vi "ILABs_RemotePanelHandler.vi"(2 "error In":errorcluster, 3 "appReference":refnum<vi>, 4 "data":string, 5 "action":string) -> (0 "errorOut":string, 1 "response":string)   [LabVIEW 2009]
panel:
  in  "Case Constant\n(See Context Help)":bool=TRUE
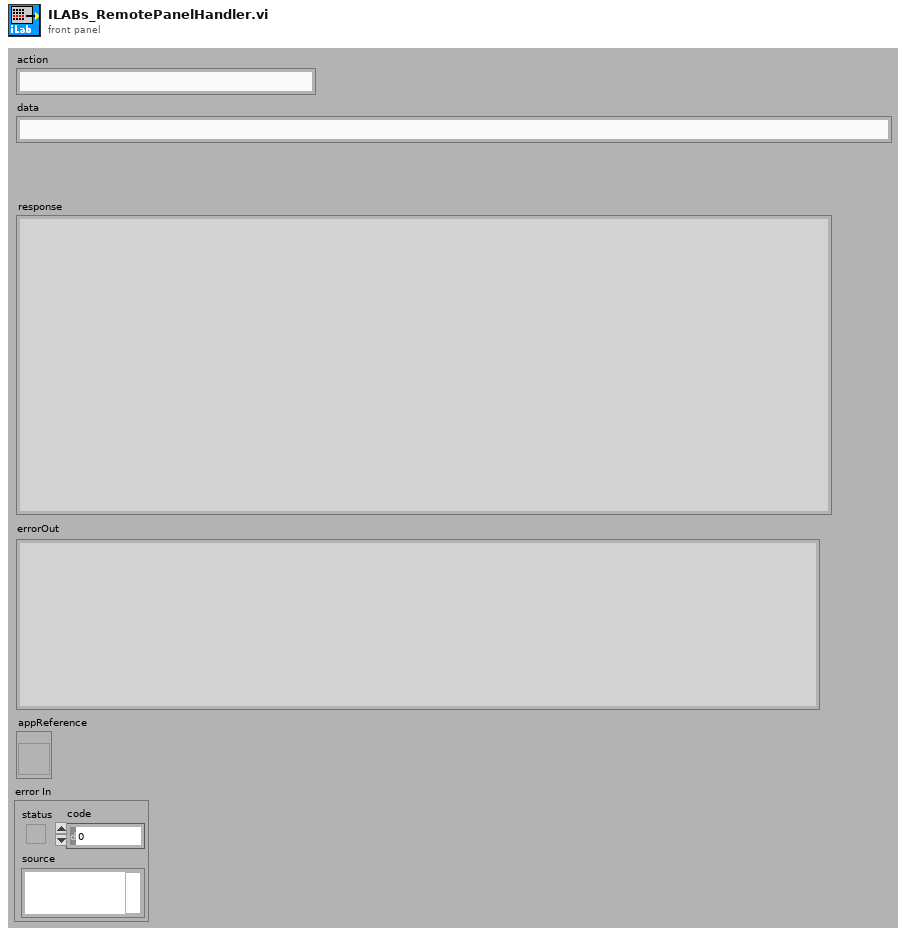
[diagram p1: front panel]
types:
  T1 = enum32{"Bad", "Idle", "Run top level", "Running"}
  T2 = typedef "LVRemotePanelConnectionsTypeDef.ctl" = cluster{"VI Name":string, "Remote":string, "UserName":string, "Port":i32, "Status":enum32{"Viewing", "Waiting For Control", "Controlling"}, "Create Time":timestamp, "Status Time":timestamp, "Control End Time":timestamp}[]
  T3 = cluster{"VI Name":string, "Remote":string, "UserName":string, "Port":i32, "Status":enum32{"Viewing", "Waiting For Control", "Controlling"}, "Create Time":timestamp, "Status Time":timestamp, "Control End Time":timestamp}
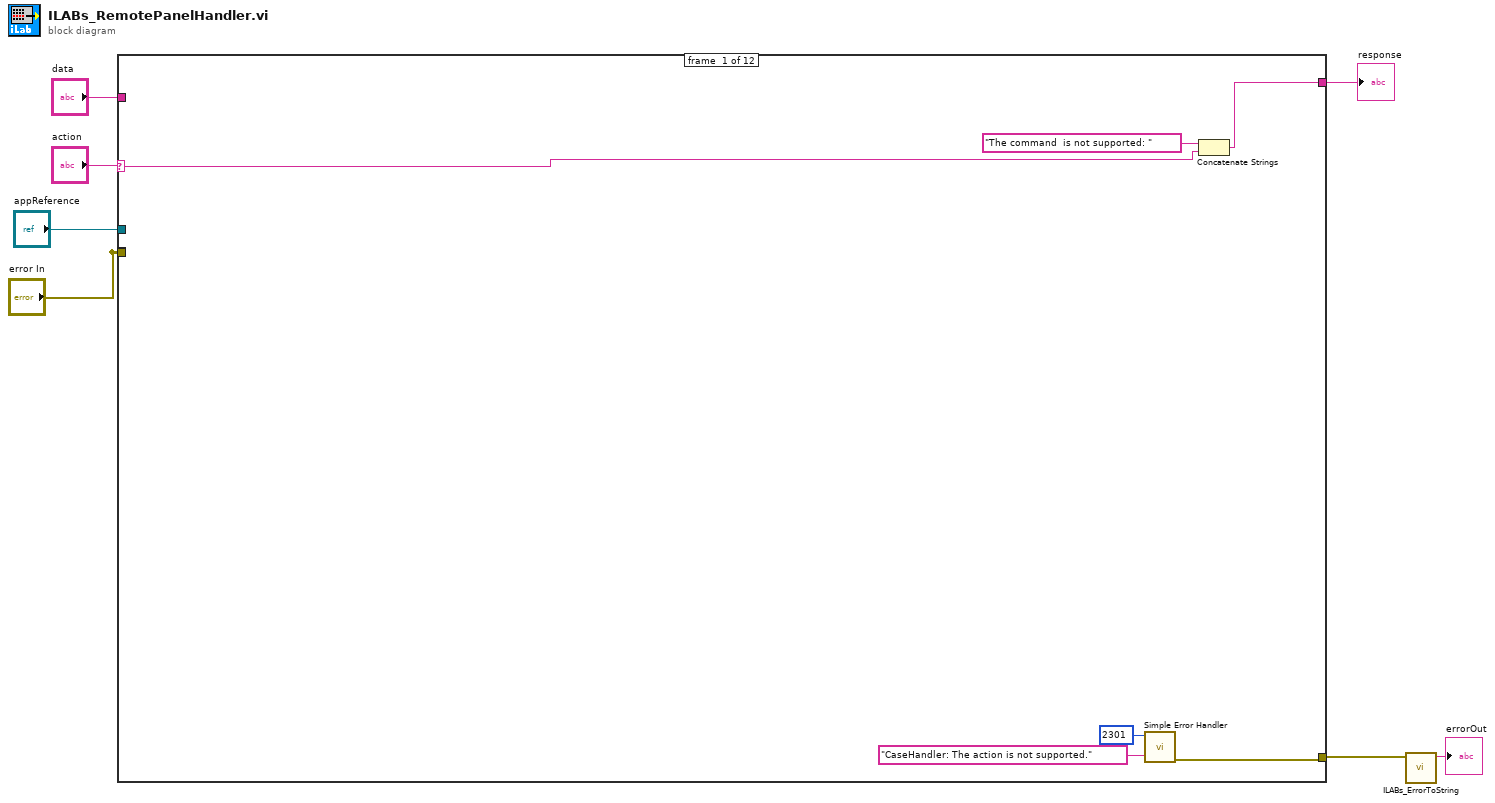
[diagram p0: block diagram]
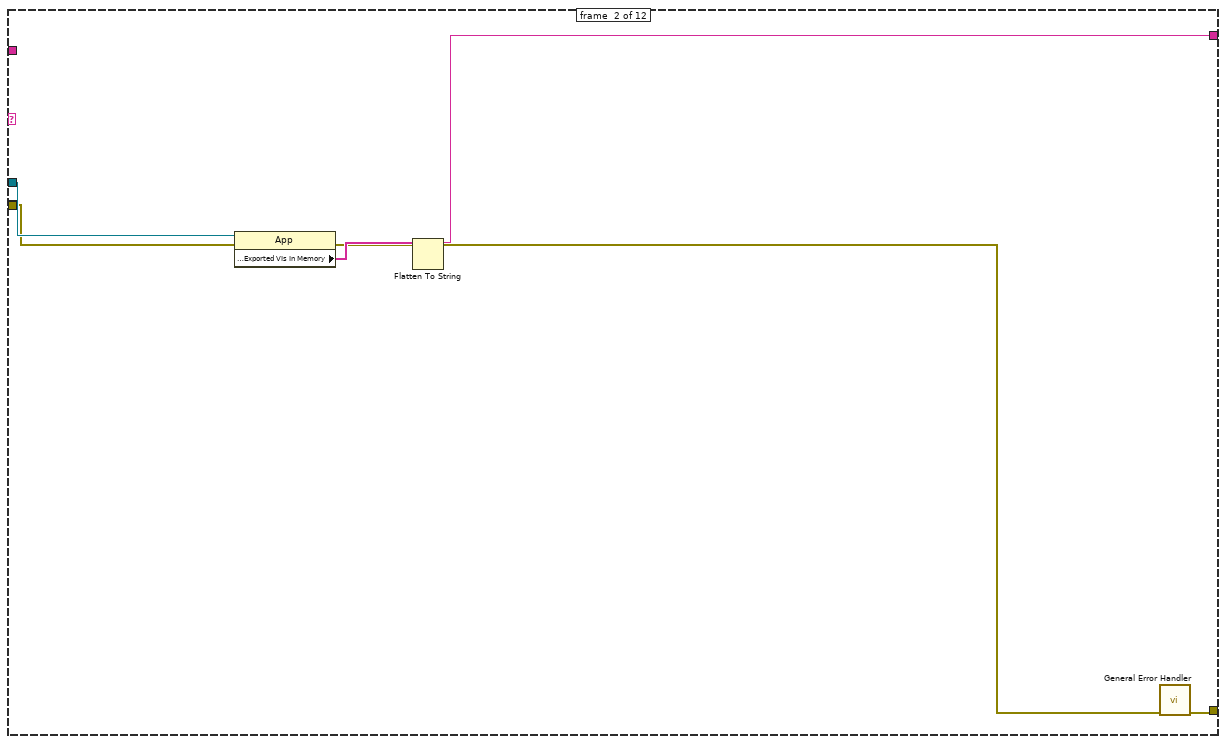
[diagram p2: hidden frame]
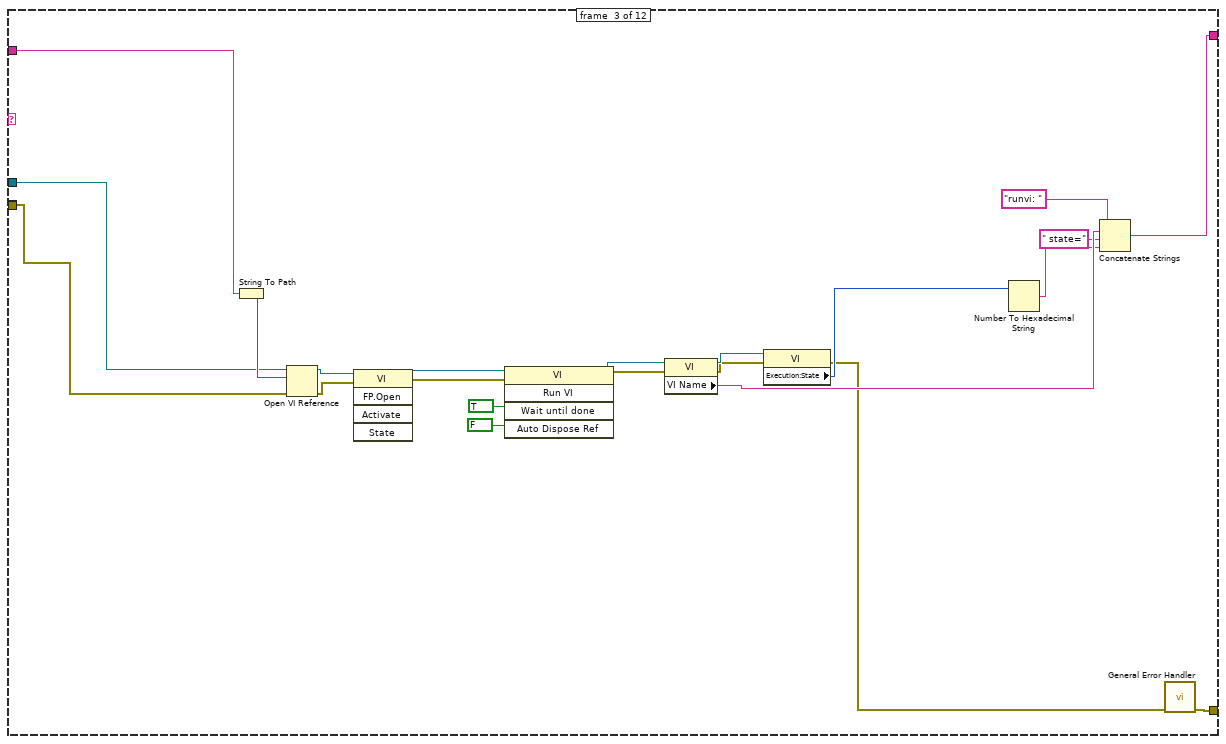
[diagram p3: hidden frame]
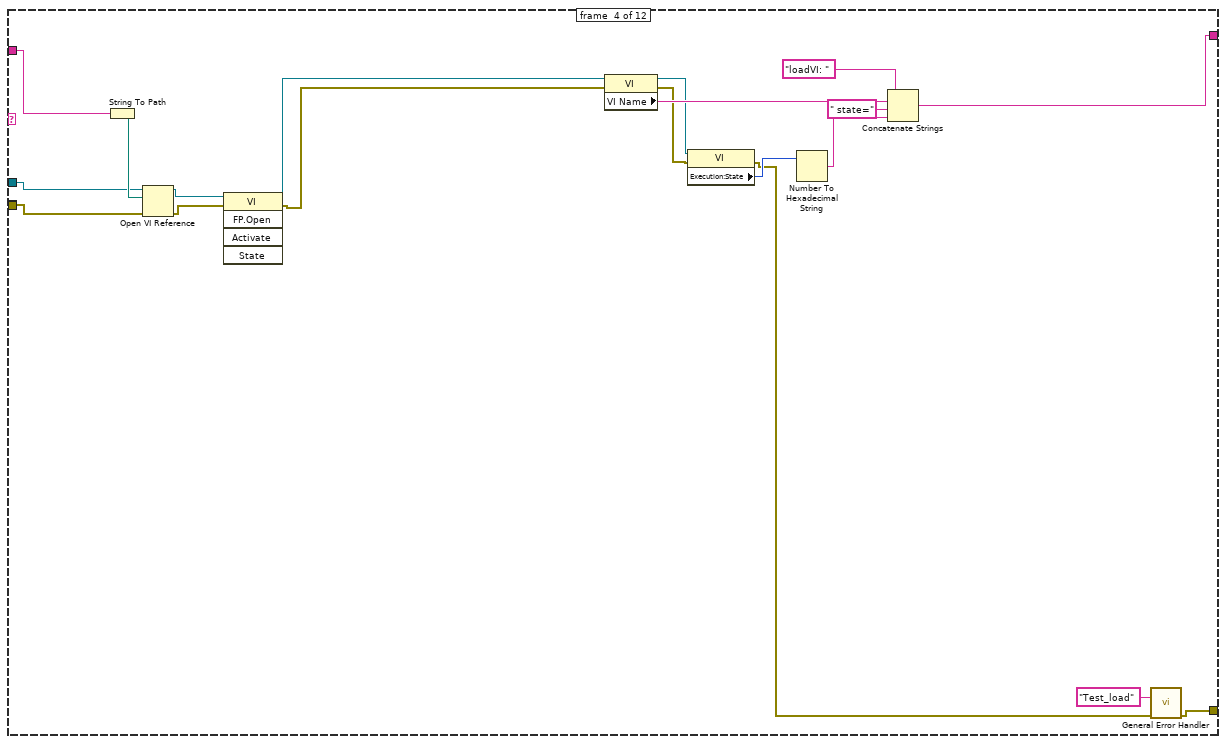
[diagram p4: hidden frame]
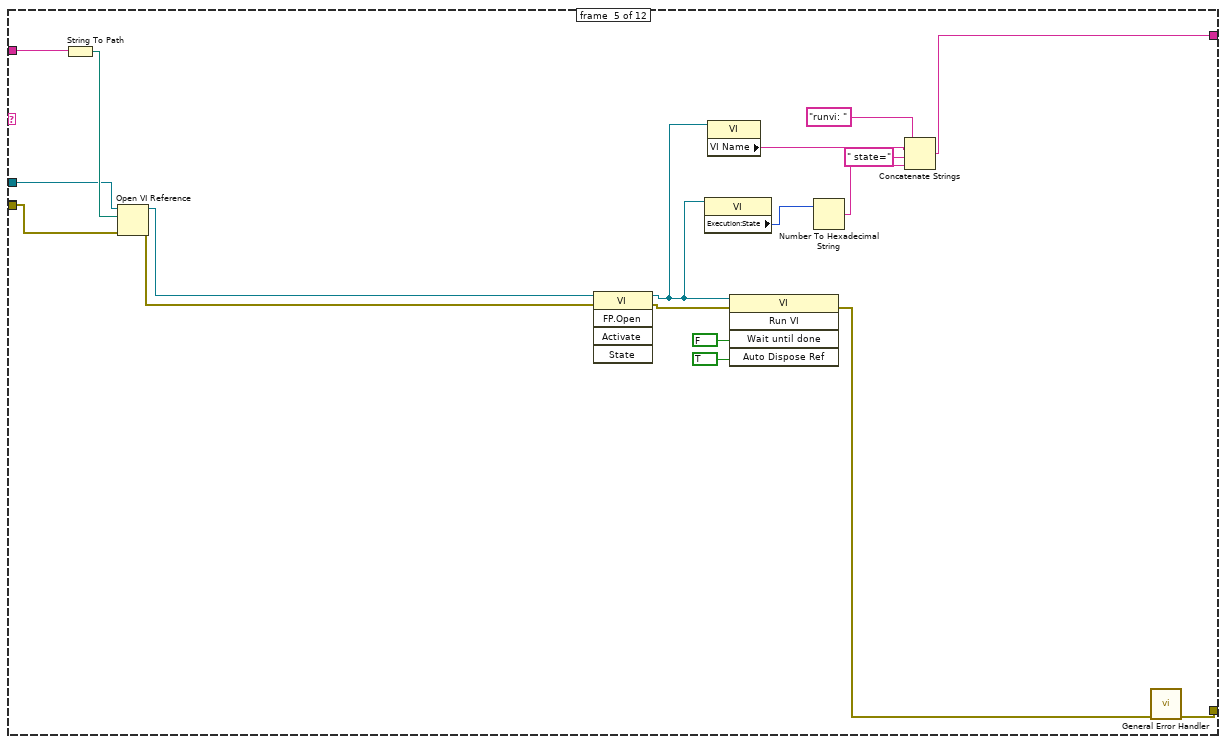
[diagram p5: hidden frame]
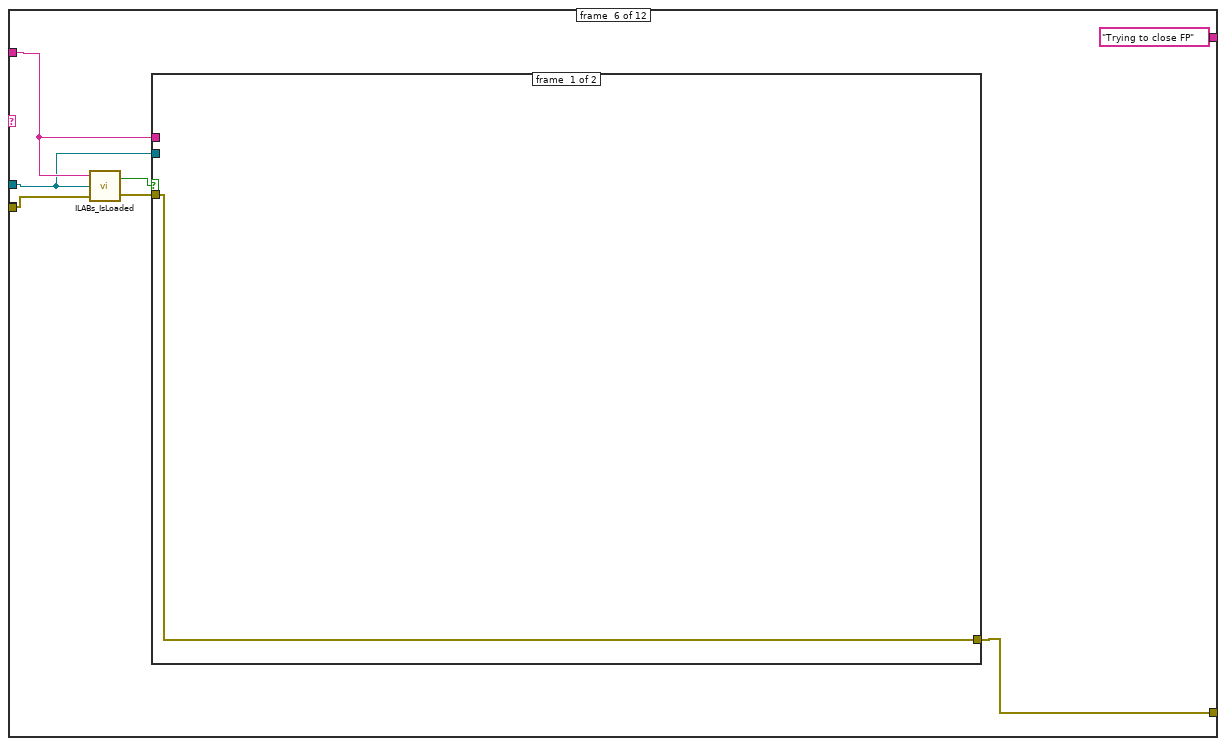
[diagram p6: hidden frame]
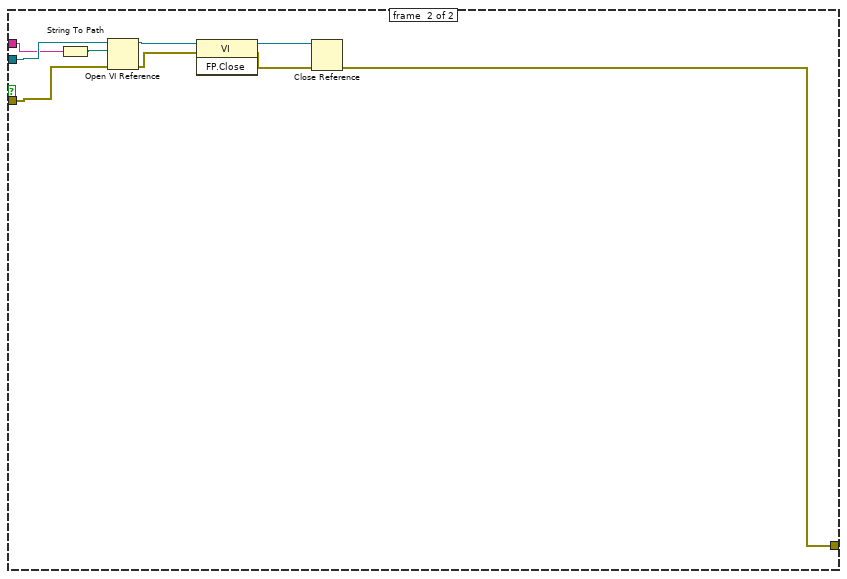
[diagram p7: hidden frame]
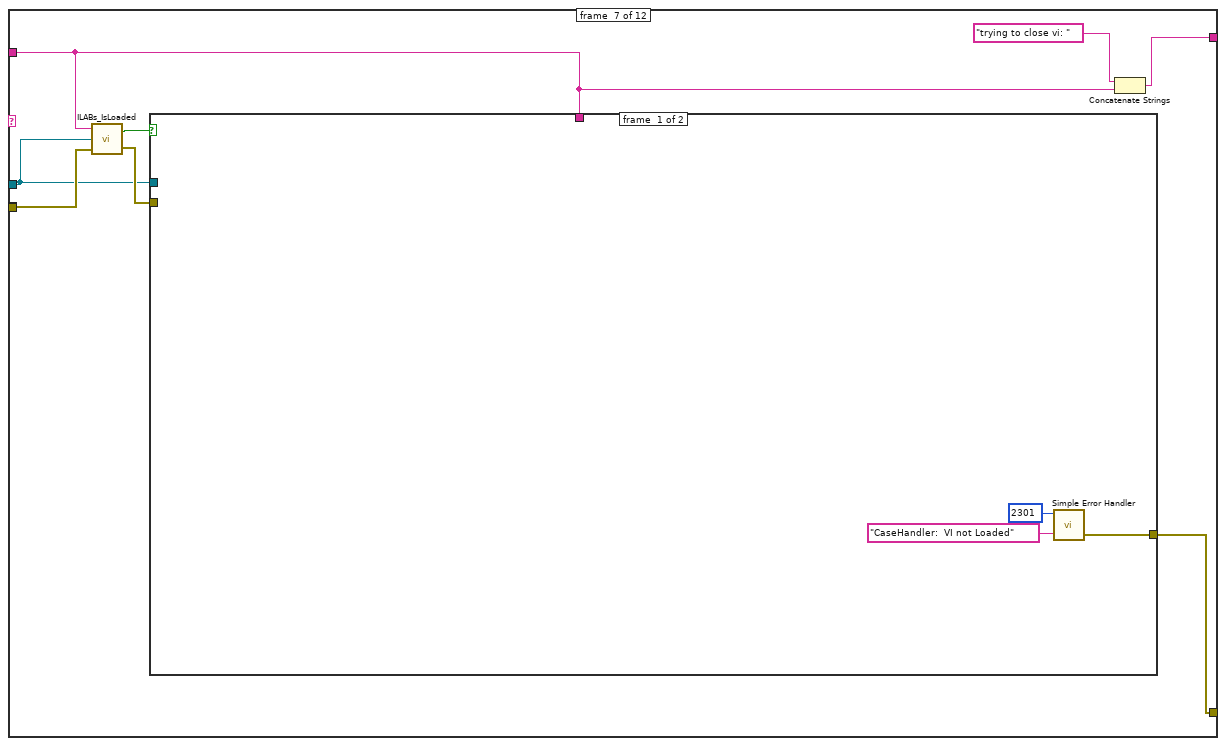
[diagram p8: hidden frame]
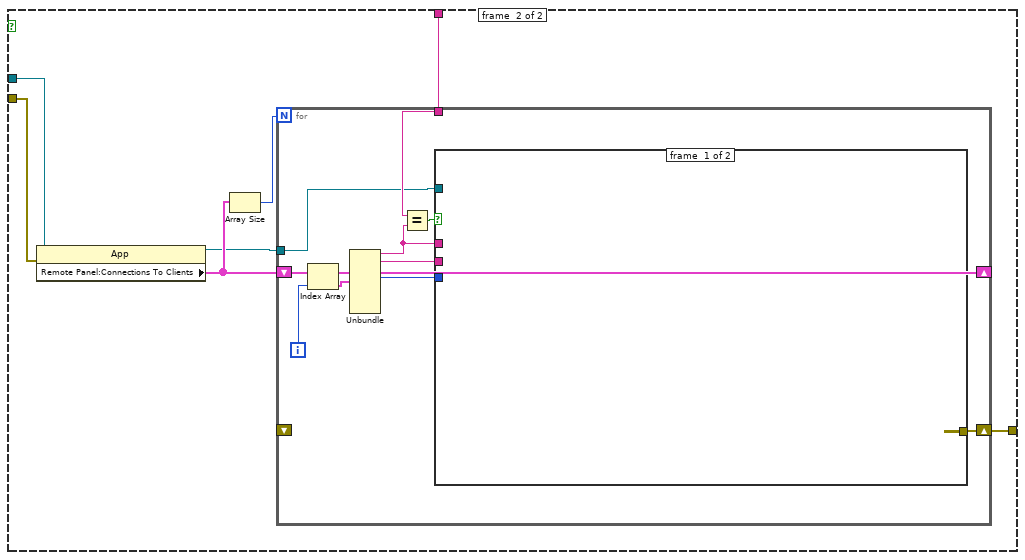
[diagram p9: hidden frame]
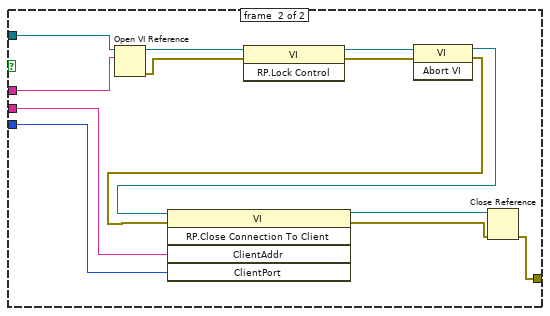
[diagram p10: hidden frame]
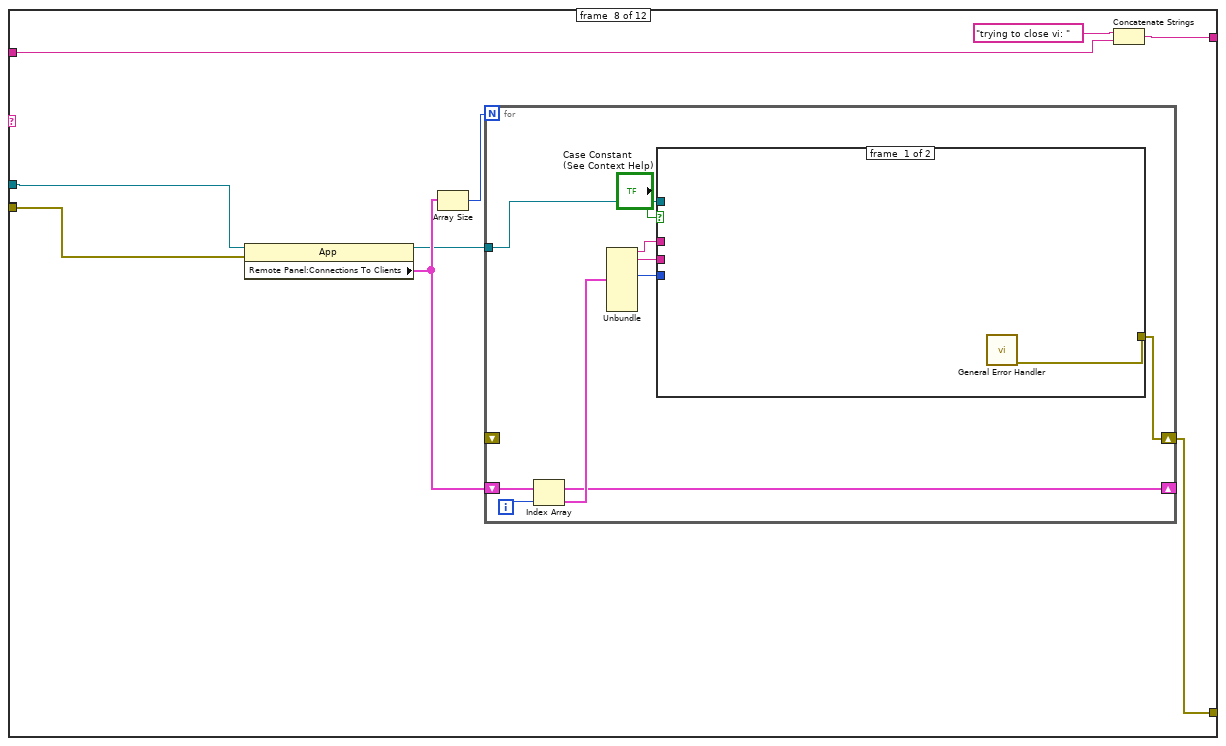
[diagram p11: hidden frame]
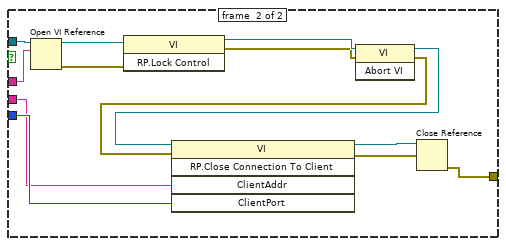
[diagram p12: hidden frame]
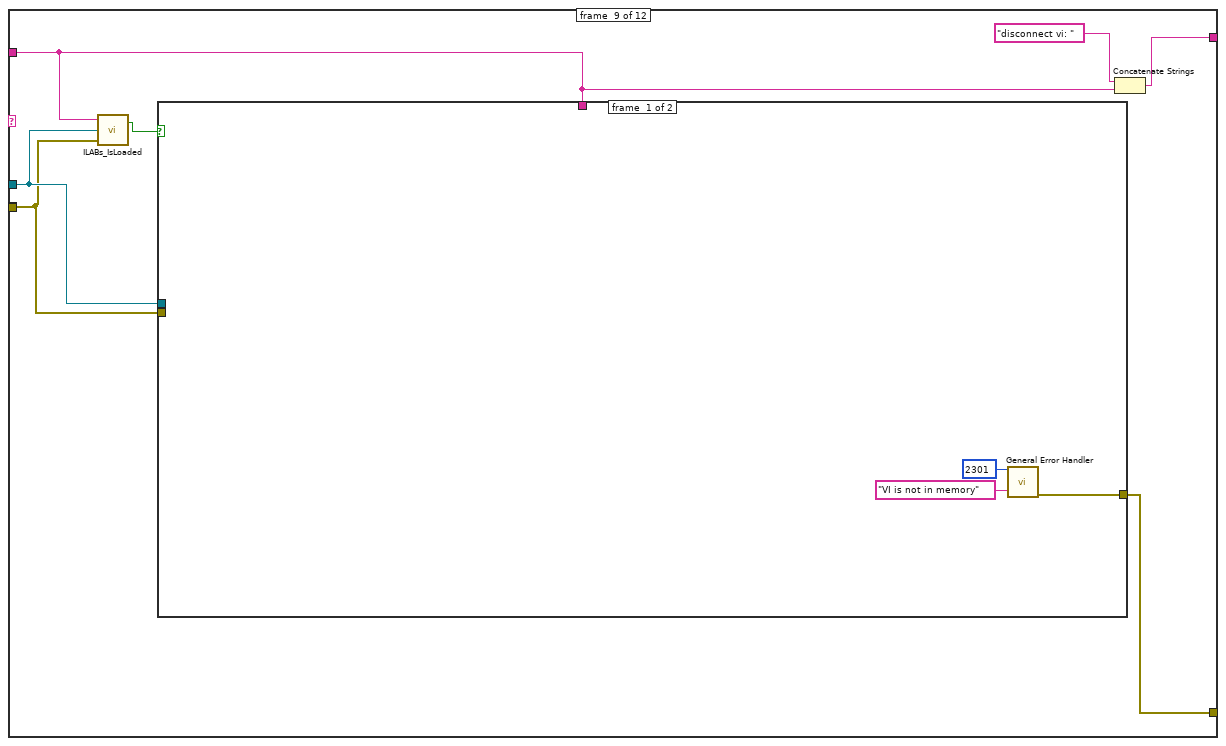
[diagram p13: hidden frame]
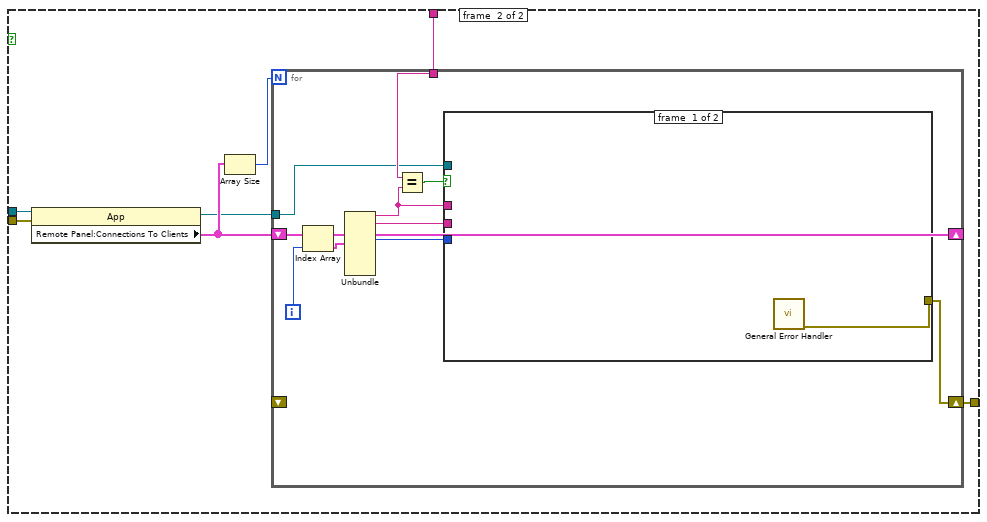
[diagram p14: hidden frame]
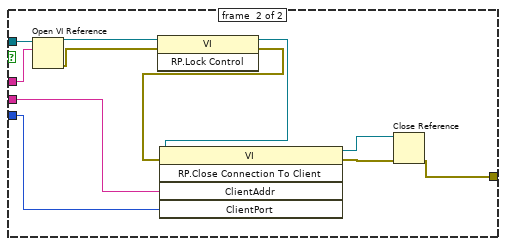
[diagram p15: hidden frame]
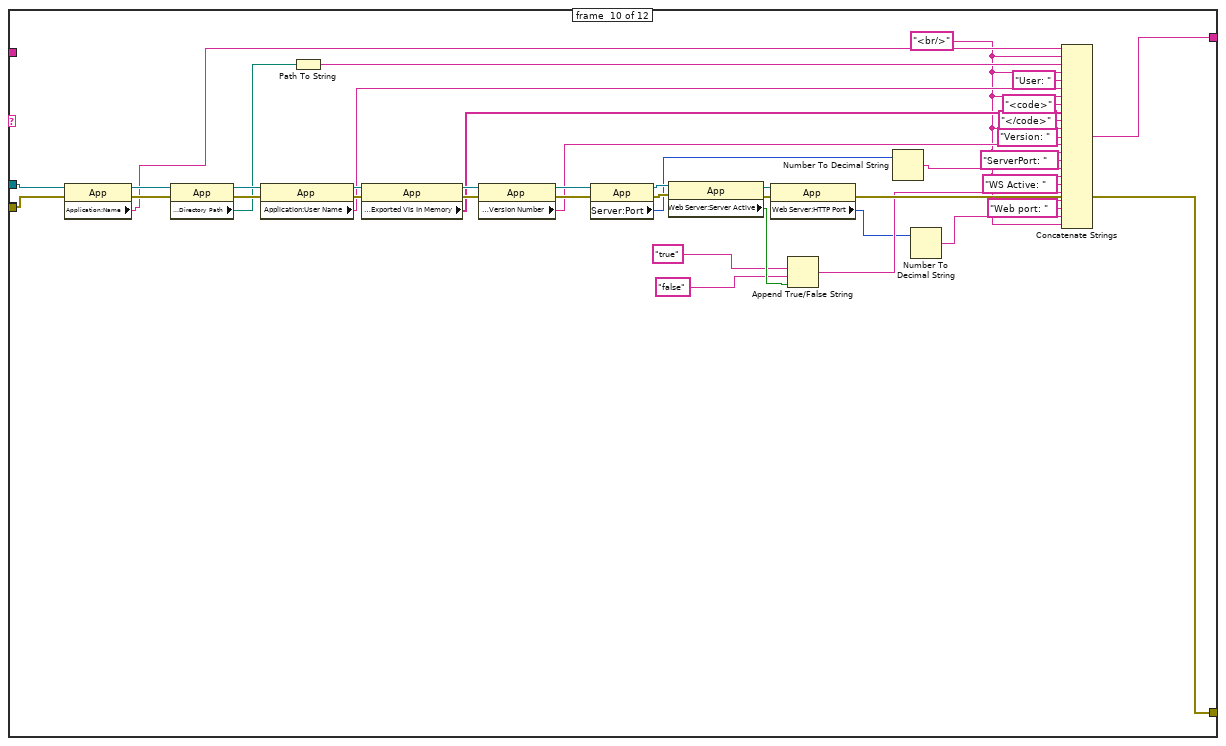
[diagram p16: hidden frame]
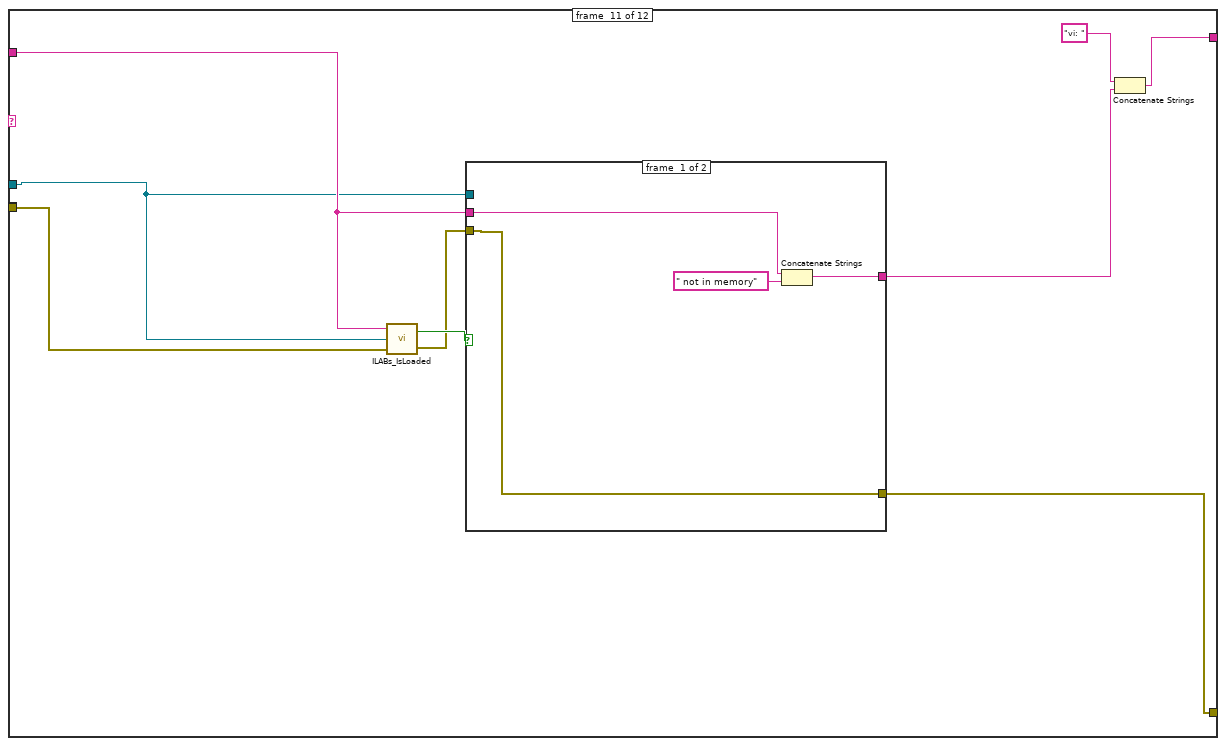
[diagram p17: hidden frame]
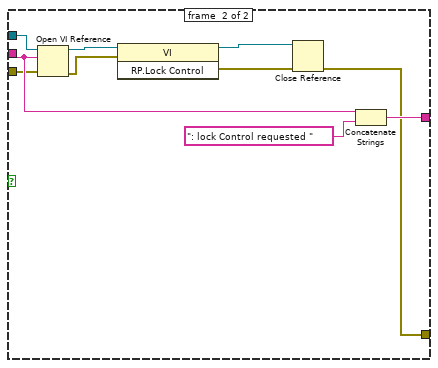
[diagram p18: hidden frame]
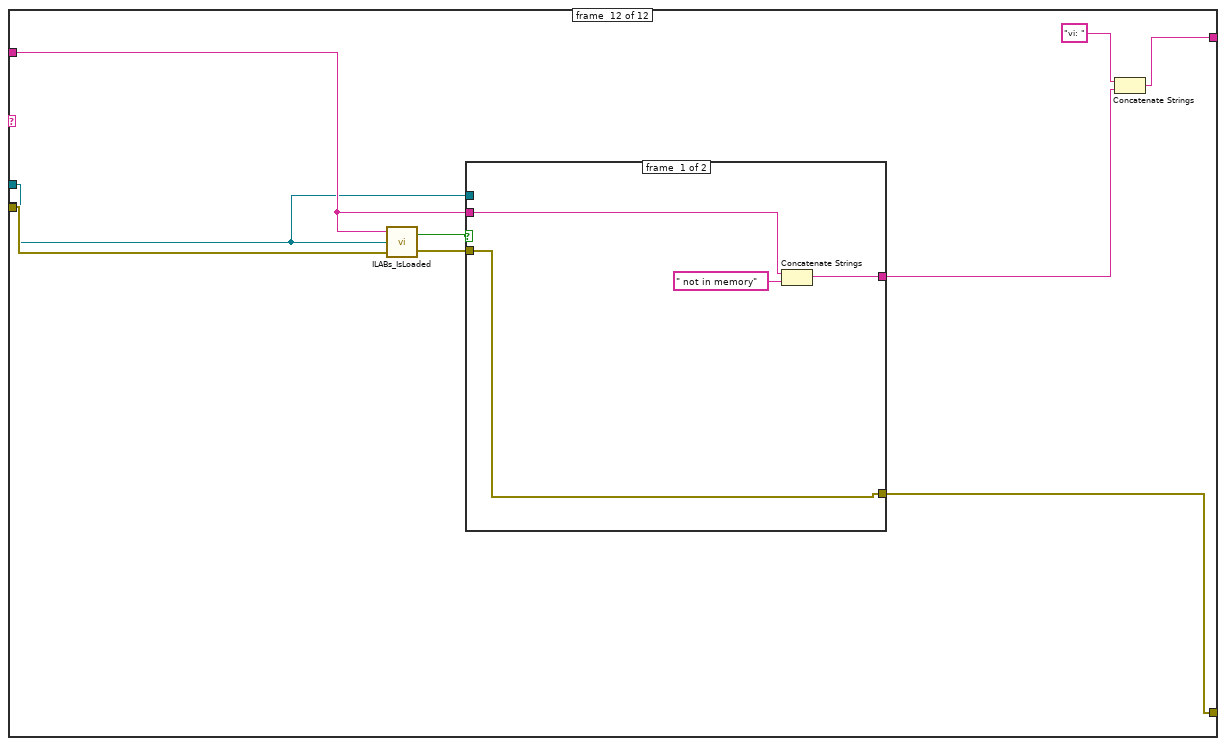
[diagram p19: hidden frame]
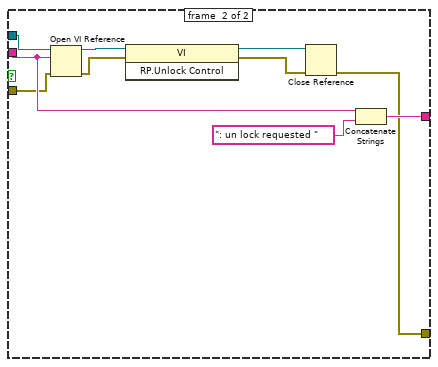
[diagram p20: hidden frame]
diagram:
  n1 = case shown="\"appstatus\"" "action" {
    selector: "action" -> [w12 _ _ _ _ _ _ _ _ _ _ _]
    tunnel: "data" -> [_ _ w37 w59 w73 w82 w100 w142 w172 _ w252 w275]
    tunnel: [w11 w19 w31 w52 w67 "Trying to close FP" ("data") w102 w141 w174 w208 w256 w279] -> w6
    tunnel: [w8 w16 w29 w51 w64 w80 w101 w140 w173 w231 w251 w274] -> w4
    tunnel: "appReference" -> [_ w15 w28 w50 w63 w81 w96 w139 w170 w247 w249 w271]
    tunnel: "error In" -> [_ w14 w27 w49 w62 w85 w98 w138 w169 w246 _ w273]
    tunnel: "error In" -> [_ _ _ _ _ _ _ _ _ _ w250 _]
    frame #0 {
      (unwired) "The" ("message")
      n2 = call <vilib>:"Simple Error Handler.vi"("error code (no error:0)"=2301, "error source (\" \")"="CaseHandler: The action is not supported." ("error source (\" \")")) -> ("error out"=w8:errorcluster)  [unwired: 2 in, 5 out]
      n3 = Concatenate Strings("The command  is not supported: " ("string"), w12) -> (w11:string)
    }
    frame #1 {
      n4 = property class="App"(reference=w15, error in=w14) -> (error out=w17:errorcluster, "Application:Exported VIs In Memory"=w18:string[])  [unwired: 1 out]
      n5 = Flatten To String(anything=w18) -> (data string=w19:string)  [unwired: 1 in, 4 out]
      n6 = call <vilib>:"General Error Handler.vi"("error in (no error)"=w17) -> ("error out"=w16:errorcluster)  [unwired: 1 in, 13 out]
    }
    frame #2 {
      n7 = String To Path(string=w37) -> (path=w38:path)
      n8 = Open VI Reference(application reference (local)=w28, vi path=w38, error in (no error)=w27) -> (vi reference=w40:refnum<vi>, error out=w39:errorcluster)  [unwired: 3 out]
      n9 = invoke class="VI" method="FP.Open"(reference=w40, error in=w39) -> (reference out=w26:refnum<vi>, error out=w25:errorcluster)  [unwired: 3 in, 3 out]
      n10 = invoke class="VI" method="Run VI"(reference=w26, error in=w25, "Wait until done"=FALSE, "Auto Dispose Ref"=TRUE) -> (reference out=w24:refnum<vi>, error out=w23:errorcluster)  [unwired: 1 in, 3 out]
      n11 = property class="VI"(reference=w24, error in=w23) -> (reference out=w22:refnum<vi>, error out=w21:errorcluster, "VI Name"=w36:string)
      n12 = property class="VI"(reference=w22, error in=w21) -> (error out=w20:errorcluster, "Execution:State"=w34:T1)  [unwired: 1 out]
      n13 = Number To Hexadecimal String(2:w34) -> (0:w33:string)  [unwired: 1 out]
      n14 = Concatenate Strings("runvi: " ("string"), w36, " state=" ("string"), w33) -> (w31:string)
      n15 = call <vilib>:"General Error Handler.vi"("error in (no error)"=w20) -> ("error out"=w29:errorcluster)  [unwired: 1 in, 13 out]
    }
    frame #3 {
      n16 = String To Path(string=w59) -> (path=w60:path)
      n17 = Open VI Reference(application reference (local)=w50, vi path=w60, error in (no error)=w49) -> (vi reference=w45:refnum<vi>, error out=w44:errorcluster)  [unwired: 3 out]
      n18 = invoke class="VI" method="FP.Open"(reference=w45, error in=w44) -> (reference out=w43:refnum<vi>, error out=w42:errorcluster)  [unwired: 3 in, 3 out]
      n19 = property class="VI"(reference=w43, error in=w42) -> (reference out=w47:refnum<vi>, error out=w48:errorcluster, "VI Name"=w57:string)
      n20 = property class="VI"(reference=w47, error in=w48) -> (error out=w46:errorcluster, "Execution:State"=w55:T1)  [unwired: 1 out]
      n21 = Number To Hexadecimal String(2:w55) -> (0:w54:string)  [unwired: 1 out]
      n22 = Concatenate Strings("loadVI: " ("string"), w57, " state=" ("string"), w54) -> (w52:string)
      n23 = call <vilib>:"General Error Handler.vi"("[error source] (\" \")"="Test_load" ("[error source] (\" \")"), "error in (no error)"=w46) -> ("error out"=w51:errorcluster)  [unwired: 1 in, 12 out]
    }
    frame #4 {
      w65 = TRUE items=["OFF", "ON", "OFF", "ON"] ("Auto Dispose Ref")
      n24 = String To Path(string=w73) -> (path=w74:path)
      n25 = Open VI Reference(application reference (local)=w63, vi path=w74, error in (no error)=w62) -> (vi reference=w77:refnum<vi>, error out=w75:errorcluster)  [unwired: 3 out]
      n26 = invoke class="VI" method="FP.Open"(reference=w77, error in=w75) -> (reference out=w72:refnum<vi>, error out=w76:errorcluster)  [unwired: 3 in, 3 out]
      n27 = property class="VI"(reference=w72) -> ("Execution:State"=w69:T1)  [unwired: 1 in, 2 out]
      n28 = property class="VI"(reference=w72) -> ("VI Name"=w71:string)  [unwired: 1 in, 2 out]
      n29 = invoke class="VI" method="Run VI"(reference=w72, error in=w76, "Wait until done"=FALSE, "Auto Dispose Ref"=w65) -> (error out=w61:errorcluster)  [unwired: 1 in, 4 out]
      n30 = Number To Hexadecimal String(2:w69) -> (0:w68:string)  [unwired: 1 out]
      n31 = Concatenate Strings("runvi: " ("string"), w71, " state=" ("string"), w68) -> (w67:string)
      n32 = call <vilib>:"General Error Handler.vi"("error in (no error)"=w61) -> ("error out"=w64:errorcluster)  [unwired: 1 in, 13 out]
    }
    frame #5 {
      n33 = call "ILABs_IsLoaded.vi"("error in (no error)"=w85, "appRef"=w81, "name"=w82) -> ("error out"=w83:errorcluster, "status"=w84:bool)
      n34 = case shown="True" w84 {
        tunnel: w83 -> [w86 w94]
        tunnel: w82 -> [_ w92]
        tunnel: w81 -> [_ w95]
        tunnel: [w86 w87] -> w80
        frame #0 {
        }
        frame #1 {
          n35 = String To Path(string=w92) -> (path=w93:path)
          n36 = Open VI Reference(application reference (local)=w95, vi path=w93, error in (no error)=w94) -> (vi reference=w91:refnum<vi>, error out=w90:errorcluster)  [unwired: 3 out]
          n37 = invoke class="VI" method="FP.Close"(reference=w91, error in=w90) -> (reference out=w89:refnum<vi>, error out=w88:errorcluster)  [unwired: 1 in, 1 out]
          n38 = Close Reference(reference=w89, error in (no error)=w88) -> (error out=w87:errorcluster)
        }
      }
    }
    frame #6 {
      n39 = call "ILABs_IsLoaded.vi"("error in (no error)"=w98, "appRef"=w96, "name"=w100) -> ("error out"=w97:errorcluster, "status"=w99:bool)
      n40 = case shown="True" w99 {
        tunnel: [w106 w111] -> w101
        tunnel: w100 -> [_ w110]
        tunnel: w97 -> [_ w108]
        tunnel: w96 -> [_ w109]
        frame #0 {
          n41 = call <vilib>:"Simple Error Handler.vi"("error code (no error:0)"=2301, "error source (\" \")"="CaseHandler:  VI not Loaded" ("error source (\" \")")) -> ("error out"=w106:errorcluster)  [unwired: 2 in, 5 out]
        }
        frame #1 {
          n42 = property class="App"(reference=w109, error in=w108) -> (reference out=w107:refnum<vi>, "Remote Panel:Connections To Clients"=w112:T2)  [unwired: 1 out]
          n43 = Array Size(array=w112) -> (size(s)=w113:i32)
          n44 = for {
            N: w113 -> [_]
            shift-right: [w115] -> _
            shift-left: w112 -> [w115]
            tunnel: w110 -> [w121]
            shift-right: [w117] -> w111
            shift-left: _ -> [_]
            tunnel: w107 -> [w114]
            i -> [w123]
            n45 = Index Array(array=w115, index=w123) -> (element=w122:T3)
            n46 = Unbundle(w122) -> ("VI Name"=w116:string, "Remote"=w118:string, "Port"=w119:i32)  [unwired: 5 out]
            n47 = Equal?(x=w121, y=w116) -> (x = y?=w120:bool)
            n48 = case shown="True" w120 {
              tunnel: w119 -> [_ w136]
              tunnel: w118 -> [_ w135]
              tunnel: [_ w134] -> w117
              tunnel: w116 -> [_ w133]
              tunnel: w114 -> [_ w124]
              frame #0 {
              }
              frame #1 {
                n49 = Open VI Reference(application reference (local)=w124, vi path=w133) -> (vi reference=w132:refnum<vi>, error out=w131:errorcluster)  [unwired: 1 in, 3 out]
                n50 = invoke class="VI" method="RP.Lock Control"(reference=w132, error in=w131) -> (reference out=w130:refnum<vi>, error out=w129:errorcluster)  [unwired: 1 in, 1 out]
                n51 = invoke class="VI" method="Abort VI"(reference=w130, error in=w129) -> (reference out=w126:refnum<vi>, error out=w128:errorcluster)  [unwired: 1 in, 1 out]
                n52 = invoke class="VI" method="RP.Close Connection To Client"(reference=w126, error in=w128, "ClientAddr"=w135, "ClientPort"=w136) -> (reference out=w125:refnum<vi>, error out=w127:errorcluster)  [unwired: 1 in, 3 out]
                n53 = Close Reference(reference=w125, error in (no error)=w127) -> (error out=w134:errorcluster)
              }
            }
          }
        }
      }
      n54 = Concatenate Strings("trying to close vi: " ("data"), w100) -> (w102:string)
    }
    frame #7 {
      n55 = property class="App"(reference=w139, error in=w138) -> (reference out=w137:refnum<vi>, "Remote Panel:Connections To Clients"=w144:T2)  [unwired: 1 out]
      n56 = Array Size(array=w144) -> (size(s)=w145:i32)
      n57 = for {
        N: w145 -> [_]
        shift-right: [w148] -> _
        shift-left: w144 -> [w148]
        shift-right: [w150] -> w140
        shift-left: _ -> [_]
        tunnel: w137 -> [w146]
        i -> [w154]
        n58 = Index Array(array=w148, index=w154) -> (element=w153:T3)
        n59 = Unbundle(w153) -> ("VI Name"=w149:string, "Remote"=w151:string, "Port"=w152:i32)  [unwired: 5 out]
        n60 = case shown="True" "Case Constant\n(See Context Help)" {
          tunnel: w152 -> [_ w168]
          tunnel: w151 -> [_ w167]
          tunnel: [w155 w166] -> w150
          tunnel: w149 -> [_ w165]
          tunnel: w146 -> [_ w156]
          frame #0 {
            n61 = call <vilib>:"General Error Handler.vi"() -> ("error out"=w155:errorcluster)  [unwired: 2 in, 13 out]
          }
          frame #1 {
            n62 = Open VI Reference(application reference (local)=w156, vi path=w165) -> (vi reference=w160:refnum<vi>, error out=w159:errorcluster)  [unwired: 1 in, 3 out]
            n63 = invoke class="VI" method="RP.Lock Control"(reference=w160, error in=w159) -> (reference out=w158:refnum<vi>, error out=w157:errorcluster)  [unwired: 1 in, 1 out]
            n64 = invoke class="VI" method="Abort VI"(reference=w158, error in=w157) -> (reference out=w161:refnum<vi>, error out=w162:errorcluster)  [unwired: 1 in, 1 out]
            n65 = invoke class="VI" method="RP.Close Connection To Client"(reference=w161, error in=w162, "ClientAddr"=w167, "ClientPort"=w168) -> (reference out=w164:refnum<vi>, error out=w163:errorcluster)  [unwired: 1 in, 3 out]
            n66 = Close Reference(reference=w164, error in (no error)=w163) -> (error out=w166:errorcluster)
          }
        }
      }
      n67 = Concatenate Strings("trying to close vi: " ("data"), w142) -> (w141:string)
    }
    frame #8 {
      n68 = call "ILABs_IsLoaded.vi"("error in (no error)"=w169, "appRef"=w170, "name"=w172) -> ("status"=w171:bool)  [unwired: 1 out]
      n69 = case shown="True" w171 {
        tunnel: [w178 w183] -> w173
        tunnel: w172 -> [_ w182]
        tunnel: w170 -> [_ w181]
        tunnel: w169 -> [_ w180]
        frame #0 {
          n70 = call <vilib>:"General Error Handler.vi"("[error code] (0)"=2301, "[error source] (\" \")"="VI is not in memory" ("[error source] (\" \")")) -> ("error out"=w178:errorcluster)  [unwired: 2 in, 11 out]
        }
        frame #1 {
          n71 = property class="App"(reference=w181, error in=w180) -> (reference out=w179:refnum<vi>, "Remote Panel:Connections To Clients"=w184:T2)  [unwired: 1 out]
          n72 = Array Size(array=w184) -> (size(s)=w185:i32)
          n73 = for {
            N: w185 -> [_]
            shift-right: [w187] -> _
            shift-left: w184 -> [w187]
            tunnel: w182 -> [w193]
            shift-right: [w189] -> w183
            shift-left: _ -> [_]
            tunnel: w179 -> [w186]
            i -> [w195]
            n74 = Index Array(array=w187, index=w195) -> (element=w194:T3)
            n75 = Unbundle(w194) -> ("VI Name"=w188:string, "Remote"=w190:string, "Port"=w191:i32)  [unwired: 5 out]
            n76 = Equal?(x=w193, y=w188) -> (x = y?=w192:bool)
            n77 = case shown="True" w192 {
              tunnel: w191 -> [_ w207]
              tunnel: w190 -> [_ w206]
              tunnel: [w196 w197] -> w189
              tunnel: w188 -> [_ w205]
              tunnel: w186 -> [_ w200]
              frame #0 {
                n78 = call <vilib>:"General Error Handler.vi"() -> ("error out"=w196:errorcluster)  [unwired: 2 in, 13 out]
              }
              frame #1 {
                n79 = Open VI Reference(application reference (local)=w200, vi path=w205) -> (vi reference=w204:refnum<vi>, error out=w201:errorcluster)  [unwired: 1 in, 3 out]
                n80 = invoke class="VI" method="RP.Lock Control"(reference=w204, error in=w201) -> (reference out=w203:refnum<vi>, error out=w202:errorcluster)  [unwired: 1 in, 1 out]
                n81 = invoke class="VI" method="RP.Close Connection To Client"(reference=w203, error in=w202, "ClientAddr"=w206, "ClientPort"=w207) -> (reference out=w198:refnum<vi>, error out=w199:errorcluster)  [unwired: 1 in, 3 out]
                n82 = Close Reference(reference=w198, error in (no error)=w199) -> (error out=w197:errorcluster)
              }
            }
          }
        }
      }
      n83 = Concatenate Strings("disconnect vi: " ("data"), w172) -> (w174:string)
    }
    frame #9 {
      w209 = "<br/>" ("string")
      n84 = property class="App"(reference=w247, error in=w246) -> (reference out=w245:refnum<vi>, error out=w240:errorcluster, "Application:Name"=w230:string)
      n85 = property class="App"(reference=w245, error in=w240) -> (reference out=w244:refnum<vi>, error out=w239:errorcluster, "Application:Directory Path"=w228:path)
      n86 = property class="App"(reference=w244, error in=w239) -> (reference out=w243:refnum<vi>, error out=w238:errorcluster, "Application:User Name"=w226:string)
      n87 = Path To String(path=w228) -> (string=w229:string)
      n88 = property class="App"(reference=w243, error in=w238) -> (reference out=w242:refnum<vi>, error out=w237:errorcluster, "Application:Exported VIs In Memory"=w224:string[])
      n89 = property class="App"(reference=w242, error in=w237) -> (reference out=w241:refnum<vi>, error out=w236:errorcluster, "Application:Version Number"=w221:string)
      n90 = property class="App"(reference=w241, error in=w236) -> (reference out=w232:refnum<vi>, error out=w233:errorcluster, "Server:Port"=w218:u32)
      n91 = property class="App"(reference=w232, error in=w233) -> (reference out=w235:refnum<vi>, error out=w234:errorcluster, "Web Server:Server Active"=w216:bool)
      n92 = property class="App"(reference=w235, error in=w234) -> (error out=w231:errorcluster, "Web Server:HTTP Port"=w211:u16)  [unwired: 1 out]
      n93 = Append True/False String(1:w216, 2:"false" ("false string"), 3:"true" ("true string")) -> (0:w215:string)  [unwired: 1 out]
      n94 = Number To Decimal String(number=w218) -> (decimal integer string=w219:string)  [unwired: 1 out]
      n95 = Number To Decimal String(number=w211) -> (decimal integer string=w210:string)  [unwired: 1 out]
      n96 = Concatenate Strings(w230, w209, w229, w209, "User: " ("string"), w226, w209, "<code>" ("string"), w224, "</code>" ("string"), w209, "Version: " ("string"), w221, w209, "ServerPort: " ("string"), w219, w209, "WS Active: " ("string"), w215, w209, "Web port: " ("string"), w210, w209) -> (w208:string)
    }
    frame #10 {
      n97 = call "ILABs_IsLoaded.vi"("error in (no error)"=w250, "appRef"=w249, "name"=w252) -> ("error out"=w248:errorcluster, "status"=w253:bool)
      n98 = case shown="True" w253 {
        tunnel: w252 -> [w260 w267]
        tunnel: [w259 w268] -> w254
        tunnel: [w257 w261] -> w251
        tunnel: w249 -> [_ w265]
        tunnel: w248 -> [w257 w264]
        frame #0 {
          n99 = Concatenate Strings(w260, " not in memory" ("string")) -> (w259:string)
        }
        frame #1 {
          n100 = Open VI Reference(application reference (local)=w265, vi path=w267, error in (no error)=w264) -> (vi reference=w270:refnum<vi>, error out=w269:errorcluster)  [unwired: 3 out]
          n101 = invoke class="VI" method="RP.Lock Control"(reference=w270, error in=w269) -> (reference out=w263:refnum<vi>, error out=w262:errorcluster)  [unwired: 1 in, 1 out]
          n102 = Close Reference(reference=w263, error in (no error)=w262) -> (error out=w261:errorcluster)
          n103 = Concatenate Strings(w267, ": lock Control requested " ("string")) -> (w268:string)
        }
      }
      n104 = Concatenate Strings("vi: " ("data"), w254) -> (w256:string)
    }
    frame #11 {
      n105 = call "ILABs_IsLoaded.vi"("error in (no error)"=w273, "appRef"=w271, "name"=w275) -> ("error out"=w272:errorcluster, "status"=w276:bool)
      n106 = case shown="True" w276 {
        tunnel: w275 -> [w283 w290]
        tunnel: [w282 w291] -> w277
        tunnel: [w280 w284] -> w274
        tunnel: w272 -> [w280 w288]
        tunnel: w271 -> [_ w287]
        frame #0 {
          n107 = Concatenate Strings(w283, " not in memory" ("string")) -> (w282:string)
        }
        frame #1 {
          n108 = Open VI Reference(application reference (local)=w287, vi path=w290, error in (no error)=w288) -> (vi reference=w293:refnum<vi>, error out=w292:errorcluster)  [unwired: 3 out]
          n109 = invoke class="VI" method="RP.Unlock Control"(reference=w293, error in=w292) -> (reference out=w286:refnum<vi>, error out=w285:errorcluster)  [unwired: 1 in, 1 out]
          n110 = Close Reference(reference=w286, error in (no error)=w285) -> (error out=w284:errorcluster)
          n111 = Concatenate Strings(w290, ": un lock requested " ("string")) -> (w291:string)
        }
      }
      n112 = Concatenate Strings("vi: " ("data"), w277) -> (w279:string)
    }
  }
  "response" <- w6
  n113 = call "ILABs_ErrorToString.vi"("errorIn"=w4) -> ("errorOut"=→"errorOut":string)  [unwired: 10 out]
